vi "路径处理子VI.vi"(11 "文件名称（包括后缀）":string="调色板.png") -> (3 "添加的路径":path)   [LabVIEW 2018]
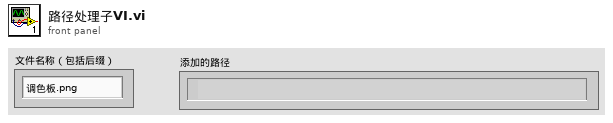
[diagram p1: front panel]
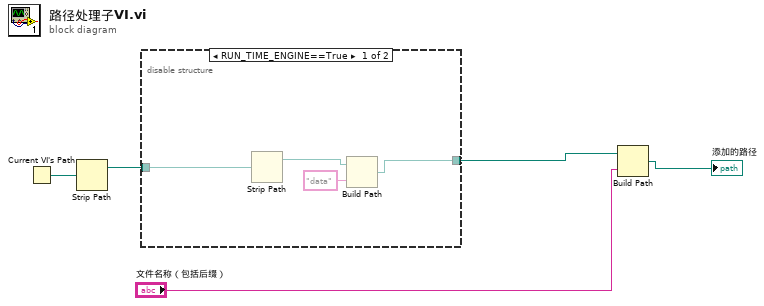
[diagram p0: block diagram]
diagram:
  n1 = Current VI's Path() -> (path=w2:path)
  n2 = Strip Path(path=w2) -> (stripped path=w1:path)  [unwired: 1 out]
  n3 = disable-structure shown="RUN_TIME_ENGINE==True" {
    disable-tunnel: [w8 w10] -> w3
    disable-tunnel: w1 -> [w6 w10]
    frame condition #0 {
      n4 = Strip Path(path=w6) -> (stripped path=w7:path)  [unwired: 1 out]
      n5 = Build Path(base path=w7, name or relative path="data") -> (appended path=w8:path)
    }
    frame condition #1 (active) {
    }
  }
  n6 = Build Path(base path=w3, name or relative path="文件名称（包括后缀）") -> (appended path=→"添加的路径":path)
